vi "Configure Digital Output Trigger.vi"(6 "Width (0)":dbl, 7 "Logic Type (0: Positive)":i32(ring) items=["Positive", "Negative"], 8 "error in (no error)":errorcluster, 9 "Digital Out Stimulus Event (\"NONE\")":string="NONE", 10 "Digital Line Trigger Source (1: line 1)":i32(ring)=1 items=["line 1"=1, "line 2"=2, "line 3"=3, "line 4"=4, "line 5"=5, "line 6"=6], 11 "VISA resource name":refnum<visa-resource-name>) -> (0 "error out":errorcluster, 3 "VISA resource name out":refnum<visa-resource-name>)   [LabVIEW 2016, in "Keithley DMM6500 DAQ6500 Series.lvlib"]
doc: "Sets the output logic of the trigger event generator to positive or negative for the specified line, describes the length of time that the trigger line is asserted for output triggers and selects the event that causes a trigger to be asserted on the digital output line."
uses:
  Keithley DMM6500 DAQ6500 Series.lvlib
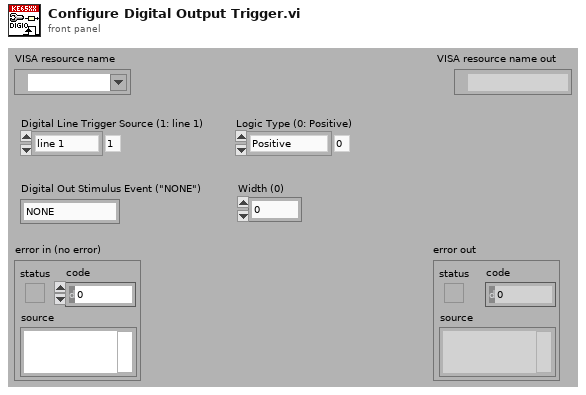
[diagram p1: front panel]
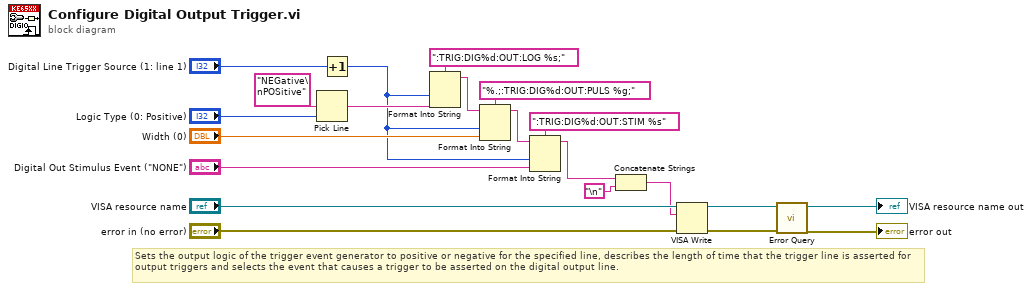
[diagram p0: block diagram]
diagram:
  # "Sets the output logic of the trigger event generator to positive or negative for the specified line, describes the length of time that the trigger line is asserted for output triggers and selects the event that causes a trigger to be asserted on the digital output line."
  n1 = Pick Line(multi-line string="NEGative\nPOSitive", line index="Logic Type (0: Positive)") -> (output string=w7:string)  [unwired: 1 in]
  n2 = Increment(x="Digital Line Trigger Source (1: line 1)") -> (x+1=w1:i32)
  n3 = Format Into String(format string=":TRIG:DIG%d:OUT:LOG %s;", w1, w7) -> (resulting string=w20:string)  [unwired: 2 in, 1 out]
  n4 = Format Into String(format string="%.;:TRIG:DIG%d:OUT:PULS %g;", initial string=w20, w1, "Width (0)") -> (resulting string=w18:string)  [unwired: 1 in, 1 out]
  n5 = Format Into String(format string=":TRIG:DIG%d:OUT:STIM %s", initial string=w18, w1, "Digital Out Stimulus Event (\"NONE\")") -> (resulting string=w3:string)  [unwired: 1 in, 1 out]
  n6 = Concatenate Strings(w3, "\n") -> (w5:string)
  n7 = VISA Write(VISA resource name="VISA resource name", write buffer=w5, error in (no error)="error in (no error)") -> (VISA resource name out=w14:refnum<visa-resource-name>, error out=w13:errorcluster)  [unwired: 1 out]
  n8 = call "Error Query.vi"("error in (no error)"=w13, "VISA resource name"=w14) -> ("error out"=→"error out":errorcluster, "VISA resource name out"=→"VISA resource name out":refnum<visa-resource-name>)  [unwired: 6 in, 2 out]
